vi "TDM2TDMSProperties.vi"(0 "tdms file in":refnum<k34>, 5 "Data Object in":refnum<k20>, 7 "group name":string, 9 "channel name":string, 11 "error in (no error)":errorcluster) -> (4 "tdms file out":refnum<k34>, 6 "Data Object out":refnum<k20>, 8 "group name out":string, 10 "channel name out":string, 15 "error out":errorcluster)   [LabVIEW 2017]
doc: "This VI copies named properties from a TDM file, channel group, or channel into corresponding channels in the target TDMS file."
uses:
  <vilib>/Platform/storage/Storage.llb/Get Property (I32).vi
  <vilib>/Platform/storage/Storage.llb/Get Property (DBL).vi
  <vilib>/Platform/storage/Storage.llb/Get Property (Time Stamp).vi
  <vilib>/Platform/storage/Storage.llb/Get Property (String).vi
  <vilib>/Platform/storage/Storage.llb/Get Property (Enum).vi
  <vilib>/Platform/storage/Storage.llb/__loadPropRefList.vi
  <vilib>/Platform/storage/Storage.llb/__loadPropString.vi
  <vilib>/Platform/storage/Storage.llb/__loadPropFloat64.vi
  <vilib>/Platform/storage/Storage.llb/__loadPropInt32.vi
  <vilib>/Platform/storage/Storage.llb/__loadPropTime.vi
  <resource>/objmgr/Storage.rc
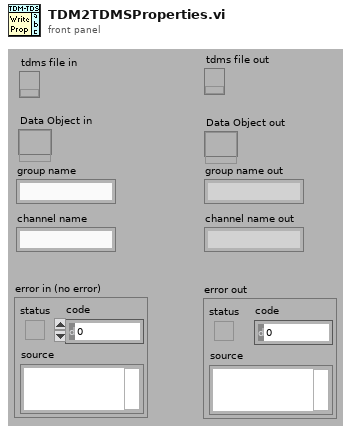
[diagram p1: front panel]
types:
  T1 = typedef "usiPropDef.ctl" = cluster{"name":string, "baseName":string, "refDataType":string, "dimensions":i32, "type":i32, "user defined":bool, "enumStrings":string[], "usiDataType":T2, "specialProp":T3, "Property Source":string, "index":i32}
  T2 = typedef "usiDataType.ctl" = enum16{"eNoTypeUsi", "eInt8Usi", "eInt16Usi", "eInt32Usi", "eInt64Usi", "eUInt8Usi", "eUInt16Usi", "eUInt32Usi", "eUInt64Usi", "eFloat32Usi", "eFloat64Usi", "- 0", "- 1", "- 2", "- 3", "- 4", "- 5", "- 6", "- 7", "- 8", "- 9", "eString8Usi", "eString16Usi", "eStringUsi", "eEnumUsi", "- 10", "- 11", "- 12", "- 13", "- 14", "eTimeUsi", "- 15", "- 16", "- 17", "- 18", "- 19", "- 20", "- 21", "- 22", "- 23", "eInstanceUsi", "eStoreUsi"}
  T3 = typedef "specialProperties.ctl" = enum16{"<Default>", "Channel Values", "AppendReplace", "ChannelFlags", "ValueFlags", "ImplicitExplicit", "InsertIndex", "ValuesCount", "ComparisonOperator", "Cluster", "DAQmx Channel"}
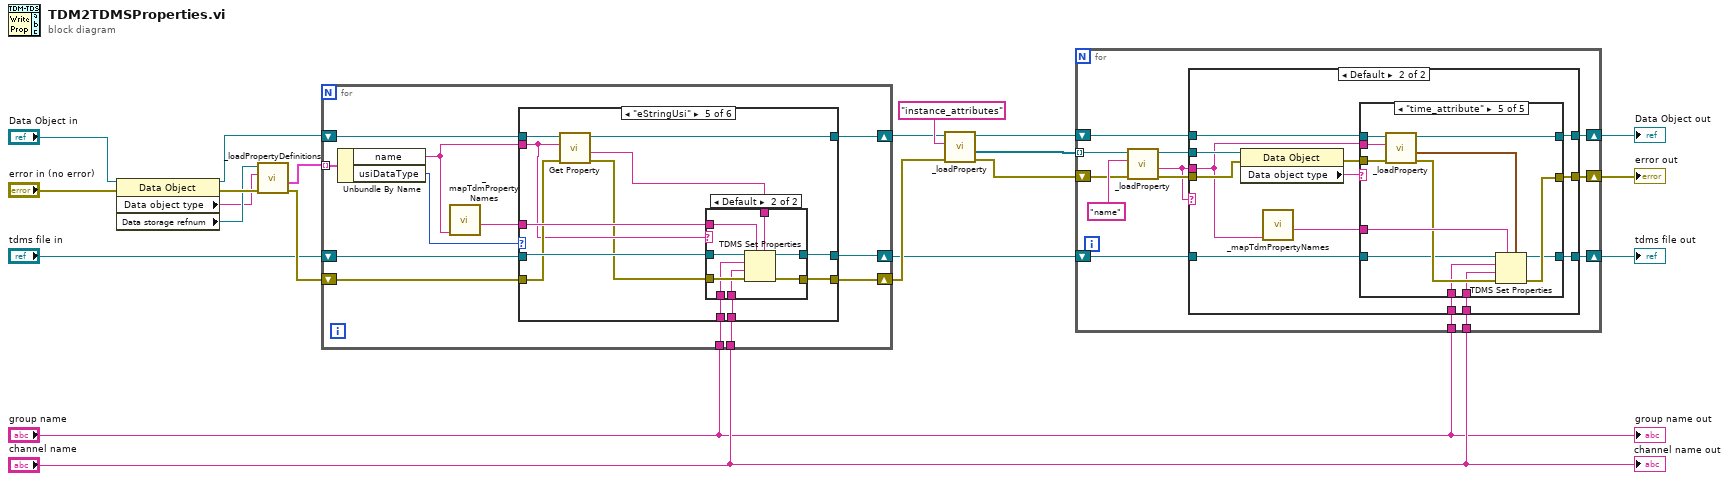
[diagram p0: block diagram]
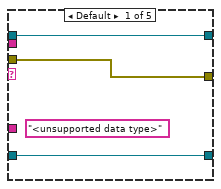
[diagram p3: hidden frame]
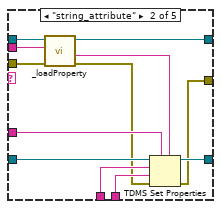
[diagram p4: hidden frame]
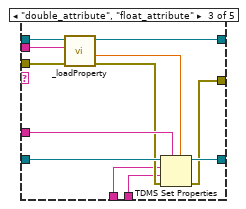
[diagram p5: hidden frame]
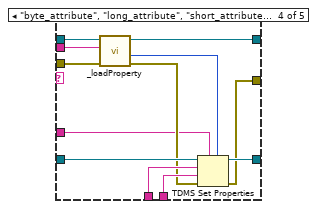
[diagram p6: hidden frame]
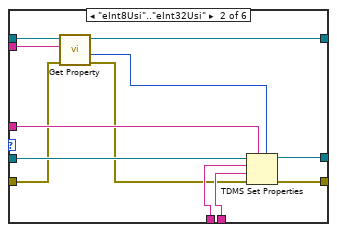
[diagram p8: hidden frame]
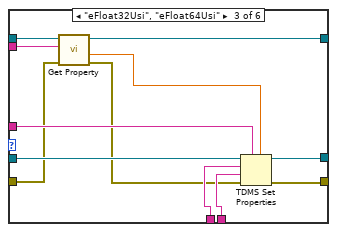
[diagram p9: hidden frame]
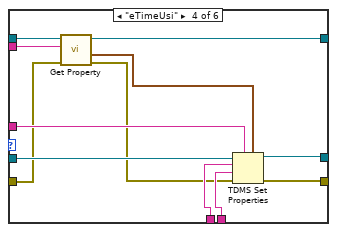
[diagram p10: hidden frame]
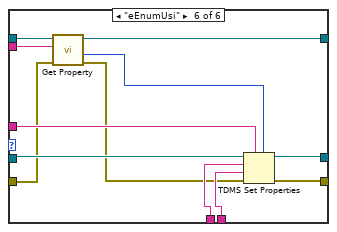
[diagram p12: hidden frame]
diagram:
  n1 = property class="Data Object"(reference="Data Object in", error in="error in (no error)") -> (reference out=w18:refnum<k20>, error out=w21:errorcluster, "Data object type"=w19:string, "Data storage refnum"=w20:refnum<k20>)
  n2 = call <vilib>:"_loadPropertyDefinitions.vi"("error in (no error)"=w21, "Object type"=w19, "storage refnum"=w20) -> ("error out"=w17:errorcluster, "PropertyDefinitions"=w16:T1[])  [unwired: 2 in, 1 out]
  n3 = for {
    shift-right: [w24] -> w8
    shift-left: w17 -> [w31]
    tunnel: w16 -> [w32] mode=indexing
    shift-right: [w26] -> w7
    shift-left: "tdms file in" -> [w29]
    shift-right: [w25] -> w10
    shift-left: w18 -> [w33]
    tunnel: "group name" -> [w23]
    tunnel: "channel name" -> [w22]
    n4 = Unbundle By Name(w32) -> ("name"=w28:string, "usiDataType"=w30:T2)
    n5 = call <vilib>:"_mapTdmPropertyNames.vi"("DNL_Name_in"=w28) -> ("DNL_Mapped_Name_out"=w27:string)  [unwired: 6 in]
    n6 = case shown="\"eStringUsi\"" w30 {
      tunnel: w28 -> [_ w48 w60 w72 w74 w106]
      tunnel: w31 -> [w34 w41 w53 w62 w78 w99]
      tunnel: w33 -> [w35 w47 w55 w67 w80 w105]
      tunnel: w29 -> [w36 w45 w59 w68 w83 w101]
      tunnel: [w36 w46 w58 w70 w84 w104] -> w26
      tunnel: w27 -> [_ w43 w56 w69 w81 w102]
      tunnel: [w35 w42 w54 w66 w79 w100] -> w25
      tunnel: [w34 w40 w52 w65 w77 w98] -> w24
      tunnel: w23 -> [_ w39 w50 w63 w76 w96]
      tunnel: w22 -> [_ w38 w51 w64 w75 w97]
      frame Default {
      }
      frame "eInt8Usi".."eInt32Usi" {
        n7 = call-poly <vilib>:"Get Property.vi"("error in (no error)"=w41, "Property name"=w48, "storage refnum"=w47) -> ("error out"=w37:errorcluster, "Value"=w44:i32, "storage refnum out"=w42:refnum<k20>)  [unwired: 6 in]
        n8 = TDMS Set Properties(5:w44, 7:w43, 8:w37, 9:w38, 10:w39, 11:w45) -> (0:w40:errorcluster, 3:w46:refnum<k34>)  [unwired: 2 out]
      }
      frame "eFloat32Usi", "eFloat64Usi" {
        n9 = call-poly <vilib>:"Get Property.vi"("error in (no error)"=w53, "Property name"=w60, "storage refnum"=w55) -> ("error out"=w49:errorcluster, "Value"=w57:dbl, "storage refnum out"=w54:refnum<k20>)  [unwired: 6 in]
        n10 = TDMS Set Properties(5:w57, 7:w56, 8:w49, 9:w51, 10:w50, 11:w59) -> (0:w52:errorcluster, 3:w58:refnum<k34>)  [unwired: 2 out]
      }
      frame "eTimeUsi" {
        n11 = call-poly <vilib>:"Get Property.vi"("error in (no error)"=w62, "Property name"=w72, "storage refnum"=w67) -> ("error out"=w61:errorcluster, "Value"=w71:timestamp, "storage refnum out"=w66:refnum<k20>)  [unwired: 6 in]
        n12 = TDMS Set Properties(5:w71, 7:w69, 8:w61, 9:w64, 10:w63, 11:w68) -> (0:w65:errorcluster, 3:w70:refnum<k34>)  [unwired: 2 out]
      }
      frame "eStringUsi" {
        n13 = call-poly <vilib>:"Get Property.vi"("error in (no error)"=w78, "Property name"=w74, "storage refnum"=w80) -> ("error out"=w73:errorcluster, "Value"=w82:string, "storage refnum out"=w79:refnum<k20>)  [unwired: 6 in]
        n14 = case shown="Default" w74 {
          tunnel: [w86 w94] -> w84
          tunnel: w83 -> [w86 w93]
          tunnel: w82 -> [_ w92]
          tunnel: w81 -> [_ w91]
          tunnel: w73 -> [w85 w90]
          tunnel: [w85 w89] -> w77
          tunnel: w76 -> [_ w88]
          tunnel: w75 -> [_ w87]
          frame "name" {
          }
          frame Default {
            n15 = TDMS Set Properties(5:w92, 7:w91, 8:w90, 9:w87, 10:w88, 11:w93) -> (0:w89:errorcluster, 3:w94:refnum<k34>)  [unwired: 2 out]
          }
        }
      }
      frame "eEnumUsi" {
        n16 = call-poly <vilib>:"Get Property.vi"("error in (no error)"=w99, "Property name"=w106, "storage refnum"=w105) -> ("error out"=w95:errorcluster, "Value"=w103:u16, "storage refnum out"=w100:refnum<k20>)  [unwired: 5 in, 1 out]
        n17 = TDMS Set Properties(5:w103, 7:w102, 8:w95, 9:w97, 10:w96, 11:w101) -> (0:w98:errorcluster, 3:w104:refnum<k34>)  [unwired: 2 out]
      }
    }
  }
  n18 = call-poly <vilib>:"_loadProperty.vi"("error in (no error)"=w8, "Property name"="instance_attributes" ("PropertyName"), "storage refnum"=w10) -> ("error out"=w2:errorcluster, "Value"=w14:refnum<k20>[], "dup storage refnum"=w9:refnum<k20>)  [unwired: 6 in]
  n19 = for {
    tunnel: w14 -> [w119] mode=indexing
    shift-right: [w116] -> w4
    shift-left: w2 -> [w117]
    shift-right: [w112] -> w3
    shift-left: w7 -> [w113]
    tunnel: "group name" -> [w111]
    tunnel: "channel name" -> [w110]
    shift-right: [w108] -> w5
    shift-left: w9 -> [w109]
    n20 = call-poly <vilib>:"_loadProperty.vi"("error in (no error)"=w117, "Property name"="name", "storage refnum"=w119) -> ("error out"=w114:errorcluster, "Value"=w107:string, "dup storage refnum"=w115:refnum<k20>)  [unwired: 6 in]
    n21 = case shown="Default" w107 {
      tunnel: [w121 w135] -> w116
      tunnel: w115 -> [_ w134]
      tunnel: w114 -> [w121 w133]
      tunnel: w107 -> [_ w130]
      tunnel: w113 -> [w120 w128]
      tunnel: [w120 w127] -> w112
      tunnel: w111 -> [_ w126]
      tunnel: w110 -> [_ w125]
      tunnel: w109 -> [w122 w124]
      tunnel: [w122 w123] -> w108
      frame "NI_ChannelLength", "NI_DataType" {
      }
      frame Default {
        n22 = property class="Data Object"(reference=w134, error in=w133) -> (error out=w131:errorcluster, "Data object type"=w132:string)  [unwired: 1 out]
        n23 = call <vilib>:"_mapTdmPropertyNames.vi"("DNL_Name_in"=w130) -> ("DNL_Mapped_Name_out"=w129:string)  [unwired: 6 in]
        n24 = case shown="\"time_attribute\"" w132 {
          tunnel: [w138 w140 w154 w164 w180] -> w135
          tunnel: w124 -> [w136 w150 w162 w174 w186]
          tunnel: w130 -> [_ w149 w161 w173 w185]
          tunnel: w131 -> [w138 w148 w160 w172 w184]
          tunnel: w129 -> [_ w144 w156 w166 w183]
          tunnel: w128 -> [w137 w146 w158 w170 w179]
          tunnel: [w137 w147 w159 w171 w178] -> w127
          tunnel: w126 -> [_ w143 w153 w169 w177]
          tunnel: w125 -> [_ w142 w152 w168 w176]
          tunnel: [w136 w139 w151 w163 w175] -> w123
          frame Default {
            (unwired) "<unsupported data type>" ("Value")
          }
          frame "string_attribute" {
            n25 = call-poly <vilib>:"_loadProperty.vi"("error in (no error)"=w148, "Property name"=w149, "storage refnum"=w150) -> ("error out"=w141:errorcluster, "Value"=w145:string, "dup storage refnum"=w139:refnum<k20>)  [unwired: 6 in]
            n26 = TDMS Set Properties(5:w145, 7:w144, 8:w141, 9:w142, 10:w143, 11:w146) -> (0:w140:errorcluster, 3:w147:refnum<k34>)  [unwired: 2 out]
          }
          frame "double_attribute", "float_attribute" {
            n27 = call-poly <vilib>:"_loadProperty.vi"("error in (no error)"=w160, "Property name"=w161, "storage refnum"=w162) -> ("error out"=w155:errorcluster, "Value"=w157:dbl, "dup storage refnum"=w151:refnum<k20>)  [unwired: 6 in]
            n28 = TDMS Set Properties(5:w157, 7:w156, 8:w155, 9:w152, 10:w153, 11:w158) -> (0:w154:errorcluster, 3:w159:refnum<k34>)  [unwired: 2 out]
          }
          frame "byte_attribute", "long_attribute", "short_attribute" {
            n29 = call-poly <vilib>:"_loadProperty.vi"("error in (no error)"=w172, "Property name"=w173, "storage refnum"=w174) -> ("error out"=w167:errorcluster, "Value"=w165:i32, "dup storage refnum"=w163:refnum<k20>)  [unwired: 6 in]
            n30 = TDMS Set Properties(5:w165, 7:w166, 8:w167, 9:w168, 10:w169, 11:w170) -> (0:w164:errorcluster, 3:w171:refnum<k34>)  [unwired: 2 out]
          }
          frame "time_attribute" {
            n31 = call-poly <vilib>:"_loadProperty.vi"("error in (no error)"=w184, "Property name"=w185, "storage refnum"=w186) -> ("error out"=w181:errorcluster, "Value"=w182:timestamp, "dup storage refnum"=w175:refnum<k20>)  [unwired: 6 in]
            n32 = TDMS Set Properties(5:w182, 7:w183, 8:w181, 9:w176, 10:w177, 11:w179) -> (0:w180:errorcluster, 3:w178:refnum<k34>)  [unwired: 2 out]
          }
        }
      }
    }
  }
  "error out" <- w4
  "Data Object out" <- w5
  "tdms file out" <- w3
  "group name out" <- "group name"
  "channel name out" <- "channel name"
